vi "Write EXCEL File.vi"(8 "错误输入":errorcluster) -> (0 "error out":errorcluster, 2 "TestDataPath":path)   [LabVIEW 2009]
uses:
  Global/Global 1.vi
panel:
  out "spreadsheet string":string
  # "Error if there is not the xls file"
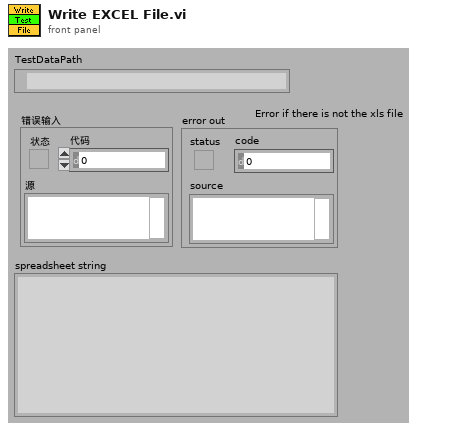
[diagram p1: front panel]
types:
  T1 = cluster{"People":string, "product  number":string, "Test time":string, "VHeatFuse_noload":string, "VHeatFuse_load":string, "VoverrideDiode":string, "Test firmware upload via X1":string, "TemperAddress":string, "Troom":string, "TLCU":string, "Adjustment factor":string, "MeasuredFreq":string, "I2C communication":string, "Light-emitting diode on Z2":string, "Battery warning/inhibit":string, "Reset by IC10":string, "External EEPROM":string, "RFID card detection and reading RFID":string, "Production parameters in internal EEPROM":string, "Current consumption in sleep mode":string, "Application and database upload":string, "Test result":string, "Table head[22]":string, "Table head[23]":string}
  T2 = enum16{"open", "replace", "create", "open or create", "replace or create", "replace or create with confirmation"}
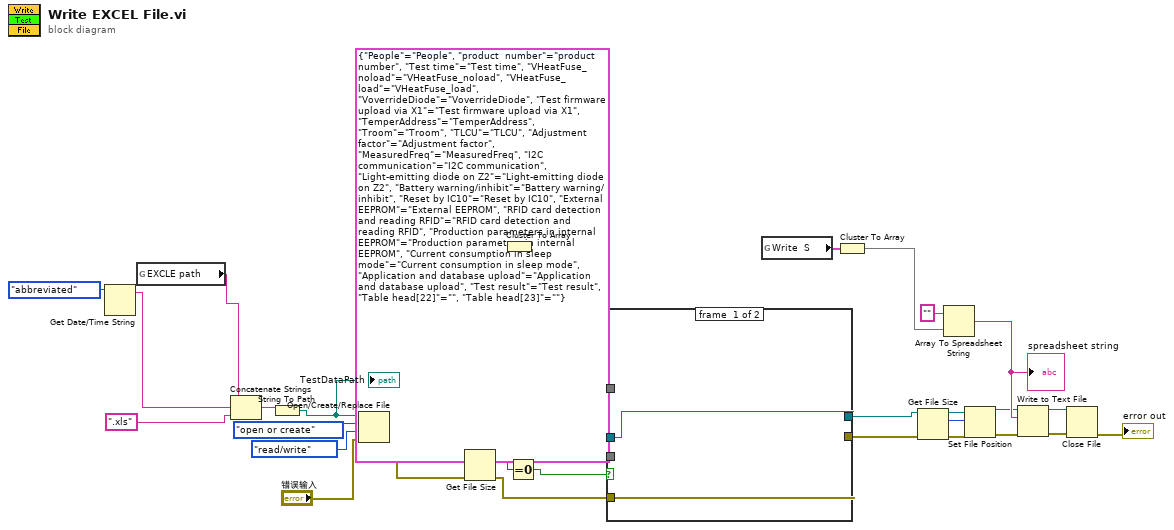
[diagram p0: block diagram]
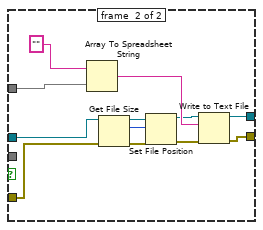
[diagram p2: hidden frame]
diagram:
  n1 = Get Date/Time String(date format (0)=enum16{"short", "long", "abbreviated"}."abbreviated") -> (date string=w22:string)  [unwired: 3 out]
  n2 = global read "Global 1.vi" "EXCLE path"() -> (w23:string)
  n3 = Concatenate Strings(w23, w22, ".xls") -> (w28:string)
  n4 = String To Path(string=w28) -> (path=w9:path)
  "TestDataPath" <- w9
  n5 = Open/Create/Replace File(file path (use dialog)=w9, error in="错误输入", operation (0:open)=T2."open or create" ("操作(0:open)"), access (0:read/write)=enum16{"read/write", "read-only", "write-only"}."read/write" ("权限(0:read/write)")) -> (refnum out=w7:refnum<file>, error out=w3:errorcluster)  [unwired: 3 out]
  n6 = Get File Size(file=w7, error in=w3) -> (refnum out=w6:refnum<file>, size (in bytes)=w5:i64, 0:w2:errorcluster)
  n7 = Cluster To Array(cluster=T1 {"People"="People", "product  number"="product  number", "Test time"="Test time", "VHeatFuse_noload"="VHeatFuse_noload", "VHeatFuse_load"="VHeatFuse_load", "VoverrideDiode"="VoverrideDiode", "Test firmware upload via X1"="Test firmware upload via X1", "TemperAddress"="TemperAddress", "Troom"="Troom", "TLCU"="TLCU", "Adjustment factor"="Adjustment factor", "MeasuredFreq"="MeasuredFreq", "I2C communication"="I2C communication", "Light-emitting diode on Z2"="Light-emitting diode on Z2", "Battery warning/inhibit"="Battery warning/inhibit", "Reset by IC10"="Reset by IC10", "External EEPROM"="External EEPROM", "RFID card detection and reading RFID"="RFID card detection and reading RFID", "Production parameters in internal EEPROM"="Production parameters in internal EEPROM", "Current consumption in sleep mode"="Current consumption in sleep mode", "Application and database upload"="Application and database upload", "Test result"="Test result", "Table head[22]"="", "Table head[23]"=""} ("Record")) -> (array=w21:string[])
  n8 = Equal To 0?(x=w5) -> (x = 0?=w4:bool)
  n9 = case shown="True" w4 {
    tunnel: w21 -> [_ _]
    tunnel: w6 -> [w33 w43]
    tunnel: w21 -> [_ w45]
    tunnel: [w33 w39] -> w15
    tunnel: [w32 w36] -> w14
    tunnel: w2 -> [w32 w34]
    frame #0 {
    }
    frame #1 {
      n10 = Array To Spreadsheet String(array=w45, 3:"" ("format string")) -> (spreadsheet string=w44:string)  [unwired: 1 out]
      n11 = Get File Size(file=w43, error in=w34) -> (refnum out=w42:refnum<file>, size (in bytes)=w41:i64, 0:w38:errorcluster)
      n12 = Set File Position(offset (in bytes) (0)=w41, refnum=w42, error in=w38) -> (refnum out=w40:refnum<file>, error out=w37:errorcluster)  [unwired: 1 out]
      n13 = Write to Text File(file (use dialog)=w40, text=w44, error in=w37) -> (refnum out=w39:refnum<file>, error out=w36:errorcluster)  [unwired: 2 out]
    }
  }
  n14 = global read "Global 1.vi" "Write  S"() -> (w25:T1)
  n15 = Cluster To Array(cluster=w25) -> (array=w18:string[])
  n16 = Get File Size(file=w15, error in=w14) -> (refnum out=w19:refnum<file>, size (in bytes)=w20:i64, 0:w13:errorcluster)
  n17 = Array To Spreadsheet String(array=w18, 3:"" ("format string")) -> (spreadsheet string=w17:string)  [unwired: 1 out]
  "spreadsheet string" <- w17
  n18 = Set File Position(offset (in bytes) (0)=w20, refnum=w19, error in=w13) -> (refnum out=w16:refnum<file>, error out=w12:errorcluster)  [unwired: 1 out]
  n19 = Write to Text File(file (use dialog)=w16, text=w17, error in=w12) -> (refnum out=w10:refnum<file>, error out=w11:errorcluster)  [unwired: 2 out]
  n20 = Close File(refnum=w10, error in=w11) -> (error out=→"error out":errorcluster)  [unwired: 1 out]
